vi "Configure Output.vi"(0 "VISA Resource Name":refnum<visa-resource-name>, 1 "Ratio Mode (0: Off)":u16(ring) items=["Off", "AUX IN 1 ", "AUX IN 2"], 2 "Offset Quantity (0: CH1, X)":u16(ring) items=["CH1, X", "CH1, R [V]", "CH1, R [dBm]", "CH2, Y"], 3 "Offset Mode (T: Automatically)":bool=TRUE, 4 "Offset Value (0.0)":dbl format="%.2f", 5 "Error In (no error)":errorcluster, 6 "Channel 2 Output (0: CH2 Display)":u16(ring) items=["CH2 Display", "Y"], 7 "Channel 1 Expand (0: X)":u16(ring) items=["X", "R [Volts rms]", "R [dBm]", "X noise"], 8 "Channel 1 Output (0: CH1 Display)":u16(ring) items=["CH1 Display", "X"], 9 "Expand CH1 (0: No Expand)":u16(ring) items=["No expand", "10", "100"], 11 "Channel 2 Expand (0: Y)":u16(ring) items=["Y", "Phi", "Y noise [Volts]"], 13 "Expand CH2 (0: No Expand)":u16(ring) items=["No expand", "10", "100"]) -> (14 "VISA Resource Name Out":refnum<visa-resource-name>, 19 "Error Out":errorcluster)   [LabVIEW 2010, in "Stanford Research 844.lvlib"]
doc: "This VI configures output."
uses:
  <instrlib>/Stanford Research 844/Stanford Research 844.lvlib
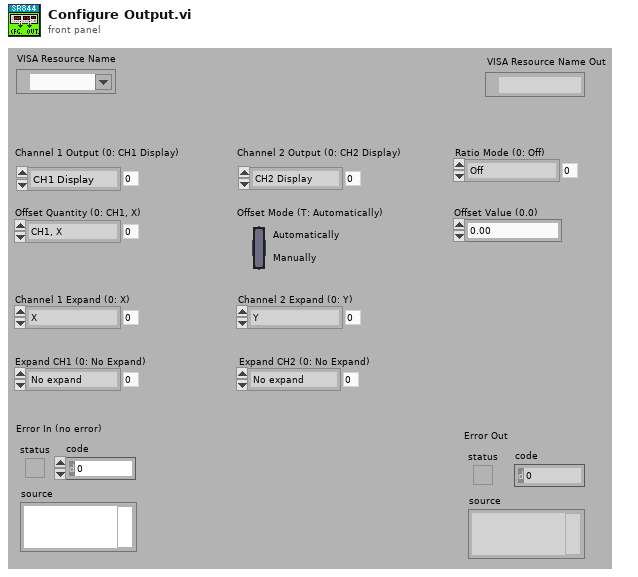
[diagram p1: front panel]
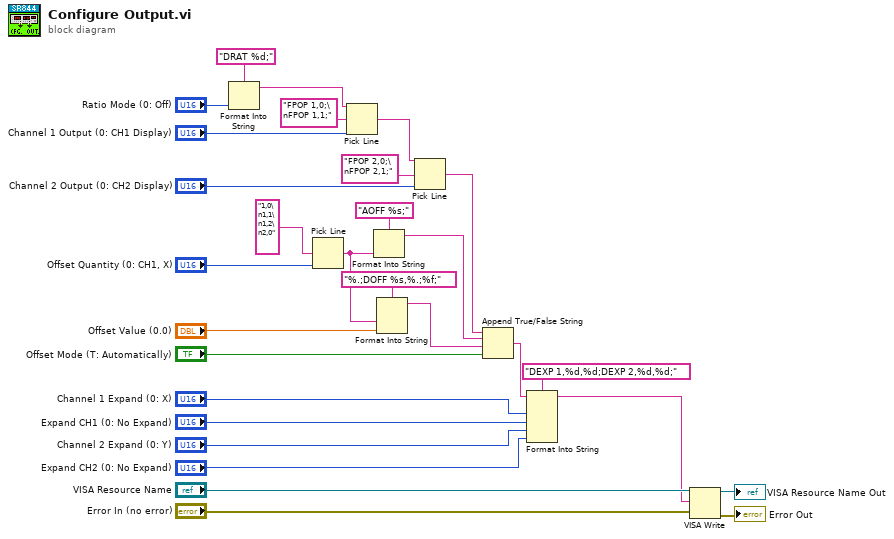
[diagram p0: block diagram]
diagram:
  n1 = Format Into String(format string="DRAT %d;", "Ratio Mode (0: Off)") -> (resulting string=w6:string)  [unwired: 2 in, 1 out]
  n2 = Pick Line(multi-line string="1,0\n1,1\n1,2\n2,0", line index="Offset Quantity (0: CH1, X)") -> (output string=w11:string)  [unwired: 1 in]
  n3 = Pick Line(string ("")=w6, multi-line string="FPOP 1,0;\nFPOP 1,1;", line index="Channel 1 Output (0: CH1 Display)") -> (output string=w2:string)
  n4 = Format Into String(format string="AOFF %s;", w11) -> (resulting string=w10:string)  [unwired: 2 in, 1 out]
  n5 = Format Into String(format string="%.;DOFF %s,%.;%f;", w11, "Offset Value (0.0)") -> (resulting string=w21:string)  [unwired: 2 in, 1 out]
  n6 = Pick Line(string ("")=w2, multi-line string="FPOP 2,0;\nFPOP 2,1;" ("true string"), line index="Channel 2 Output (0: CH2 Display)") -> (output string=w3:string)
  n7 = Append True/False String(1:"Offset Mode (T: Automatically)", 2:w21, 3:w10, 4:w3) -> (0:w17:string)
  n8 = Format Into String(format string="DEXP 1,%d,%d;DEXP 2,%d,%d;", initial string=w17, "Channel 1 Expand (0: X)", "Expand CH1 (0: No Expand)", "Channel 2 Expand (0: Y)", "Expand CH2 (0: No Expand)") -> (resulting string=w9:string)  [unwired: 1 in, 1 out]
  n9 = VISA Write(VISA resource name="VISA Resource Name", write buffer=w9, error in (no error)="Error In (no error)") -> (VISA resource name out=→"VISA Resource Name Out":refnum<visa-resource-name>, error out=→"Error Out":errorcluster)  [unwired: 1 out]
